vi "CS++RT-Main.vi"() -> ()   [LabVIEW 2014]
doc: "This is the CS++RT-Main.vi. It will launch the CS++RT-Root-Actor."
uses:
  CS++RTRoot/CS++RTRootActor.lvclass
  CSPP_LNA/CS++LNAMessage/CS++LNAMessage.lvclass
  CS++RTRoot/CS++RTRootActor.lvclass/CS++RTRootActor.ctl
  <vilib>/ActorFramework/Message Enqueuer/Message Enqueuer.lvclass/Message Enqueuer.ctl
  <vilib>/ActorFramework/Message Enqueuer/Enqueue.vi
  <vilib>/ActorFramework/Message Priority Queue/Priority Enqueue.vi
  <vilib>/ActorFramework/Stop Msg/Stop Msg.lvclass
  <vilib>/ActorFramework/Actor/Actor.lvclass
panel:
  out "Loop":i32
  in  "Stop":bool
  out "Error":errorcluster
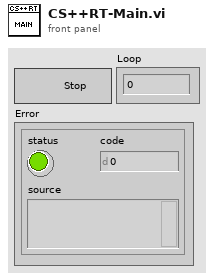
[diagram p1: front panel]
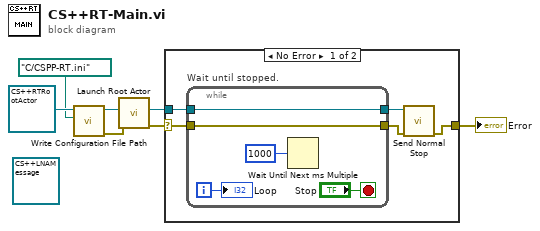
[diagram p0: block diagram]
diagram:
  (unwired) refnum<class "CS++LNAMessage.lvclass"> refnum ("CS++LNA.lvlib:CS++LNAMessage.lvclass")
  n1 = call "Write Configuration File Path.vi"("Configuration File Path"=path "C:/CSPP-RT.ini", "CS++RTRootActor in"=refnum<class "CS++RTRootActor.lvclass"> refnum ("CS++RTRoot.lvlib:CS++RTRoot.lvclass")) -> ("Error Out"=w1:errorcluster, "CS++RTRootActor out"=w3:refnum<class "CS++RTRootActor.lvclass">)  [unwired: 8 in]
  n2 = call <vilib>:"Launch Root Actor.vi"("error in (no error)"=w1, "Actor"=w3) -> ("error out"=w6:errorcluster, "Actor's Enqueuer"=w5:refnum<class "Message Enqueuer.lvclass">)  [unwired: 8 in]
  n3 = case shown="No Error" w6 {
    selector: w6 -> [w11 w18]
    tunnel: w5 -> [w12 _]
    tunnel: [w8 w18] -> w7
    frame No Error {
      n4 = while "Wait until stopped." {
        tunnel: [w17] -> w10
        tunnel: w12 -> [w17]
        tunnel: [w14] -> w9
        tunnel: w11 -> [w14]
        i -> [w13]
        stop <- "Stop" stop-if-true
        n5 = Wait Until Next ms Multiple(millisecond multiple=u32 1000) -> ()  [unwired: 1 out]
        "Loop" <- w13
      }
      n6 = call <vilib>:"Send Normal Stop.vi"("error in (no error)"=w9, "Message Enqueuer"=w10) -> ("error out"=w8:errorcluster)  [unwired: 9 in]
    }
    frame Error {
    }
  }
  "Error" <- w7
